vi "Check Settings Changed.vi"(8 "error in (no error)":errorcluster, 11 "Output Sequencer in":refnum<class "Output Sequencer.lvclass">) -> (0 "error out":errorcluster, 3 "Output Sequencer out":refnum<class "Output Sequencer.lvclass">)   [LabVIEW 2020, in "Output Sequencer.lvlib" / "Output Sequencer.lvclass"]
uses:
  Output Sequencer.lvclass
  C:/Program Files/National Instruments/LabVIEW 2024/vi.lib/FlexLogger/SDK/PluginSDK.lvlibp/PEFClasses/SDK/Plugin/Plugin.lvclass
  Output Sequencer.lvclass/Output Sequencer.ctl
  Globals/Global Strings.vi
  <vilib>/FlexLogger/SDK/PluginSDK.lvlibp/PEFClasses/SDK/Plugin/ParameterAccess/Write String.vi
  <vilib>/FlexLogger/SDK/PluginSDK.lvlibp/PEFClasses/SDK/Plugin/Plugin.lvclass
  C:/Program Files/National Instruments/LabVIEW 2024/vi.lib/FlexLogger/SDK/PluginSDK.lvlibp/PEFClasses/SDK/Processing Element/Processing Element.lvclass
  C:/Dev/GitHub/ni/niflexlogger-plugins/plugins/Output Sequencer/source/Output Sequencer/Output Sequencer/Output Sequencer.lvclass
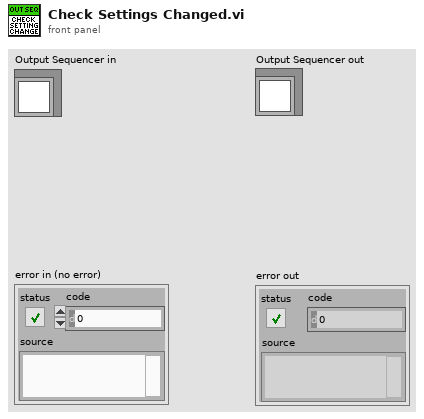
[diagram p1: front panel]
types:
  T1 = typedef "Output Sequencer.lvlib/Settings UI.lvclass/Settings.ctl" = cluster{"Plug-in Version":string, "Step Values":T2[], "Only Execute When Test Running":bool, "Reset Sequence When Test Starts":bool, "Number of Sequence Steps":i32, "Num of Analog Channels":i32, "Num of Digital Channels":i32, "Delay Before Starting Sequence":dbl, "Default Analog Values":dbl[], "Default Digital Values":bool[], "Max Iterations":u32, "Use last value when stopped":bool, "Prioritize exact values":bool, "Enable advanced step timing":bool, "Enable step conditions":bool, "Show confirmation dialogs":bool, "Start condition":string, "Enable re-triggering":bool, "Stop condition":string}
  T2 = typedef "Output Sequencer.lvlib/Settings UI.lvclass/Step Settings.ctl" = cluster{"Description":string, "Precondition":string, "Duration":dbl, "Mode":string, "Delay Between Values":dbl, "Analog Values":string[], "Digital Values":string[], "Postcondition":string, "On True":string, "On False":string}
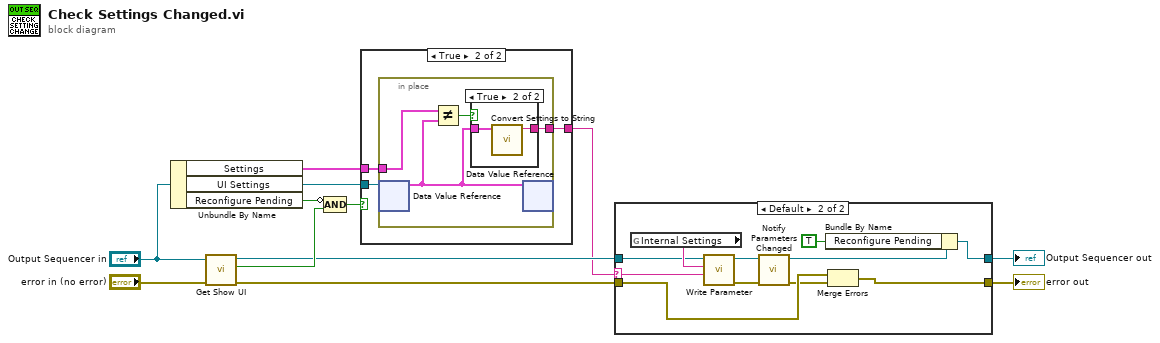
[diagram p0: block diagram]
diagram:
  n1 = Unbundle By Name("Output Sequencer in") -> ("Settings"=w7:T1, "UI Settings"=w10:refnum<data-value>, "Reconfigure Pending"=w9:bool)
  n2 = call "Get Show UI.vi"("error in (no error)"="error in (no error)", "Output Sequencer in"="Output Sequencer in") -> ("error out"=w4:errorcluster, "Show UI"=w6:bool, "Output Sequencer out"=w5:refnum<class "Output Sequencer.lvclass">)  [unwired: 7 in]
  n3 = Compound Arithmetic op=AND(invert w9, w6) -> (w8:bool)
  n4 = case shown="True" w8 {
    tunnel: w10 -> [_ w15]
    tunnel: [_ w14] -> w1
    tunnel: w7 -> [_ w13]
    frame False {
    }
    frame True {
      n5 = in-place {
        in-place-border: [w16] -> w14
        in-place-border: w13 -> [w18]
        n6 = in-place-dvr #1(w15) -> (w17:T1)  [unwired: 1 out]
        n7 = Not Equal?(x=w18, y=w17) -> (x != y?=w19:bool)
        n8 = case shown="True" w19 {
          tunnel: w17 -> [_ w21]
          tunnel: [_ w20] -> w16
          frame False {
          }
          frame True {
            n9 = call "Convert Settings to String.vi"("Settings in"=w21) -> ("String out"=w20:string)  [unwired: 9 in, 1 out]
          }
        }
        n10 = in-place-dvr #1(w17) -> ()  [unwired: 2 out]
      }
    }
  }
  n11 = case shown="Default" w1 {
    selector: w1 -> [_ w27]
    tunnel: w4 -> [w22 w26]
    tunnel: w5 -> [w23 w33]
    tunnel: [w23 w29] -> w3
    tunnel: [w22 w24] -> w2
    frame "" {
    }
    frame Default {
      n12 = global read "Global Strings.vi" "Internal Settings"() -> (w34:string)
      n13 = call-poly <vilib>:"Write Parameter.vi"("Value"=w27, "Name"=w34, "Plugin in"=w33) -> ("error out"=w31:errorcluster, "Plugin out"=w32:refnum<class "Output Sequencer.lvclass">)  [unwired: 7 in]
      n14 = call <vilib>:"Notify Parameters Changed.vi"("error in (no error)"=w31, "Plugin in"=w32) -> ("error out"=w25:errorcluster, "Plugin out"=w30:refnum<class "Output Sequencer.lvclass">)  [unwired: 8 in]
      n15 = Bundle By Name(cluster=w30, "Reconfigure Pending"=TRUE) -> (w29:refnum<class "Output Sequencer.lvclass">)
      n16 = Merge Errors(w26, w25) -> (w24:errorcluster)
    }
  }
  "Output Sequencer out" <- w3
  "error out" <- w2
